vi "9202_conversions.vi"(11 "data":dbl[](array[numeric])) -> (3 "Array":dbl[](array[numeric]))   [LabVIEW 2019]
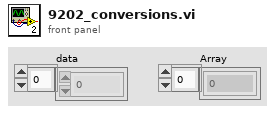
[diagram p1: front panel]
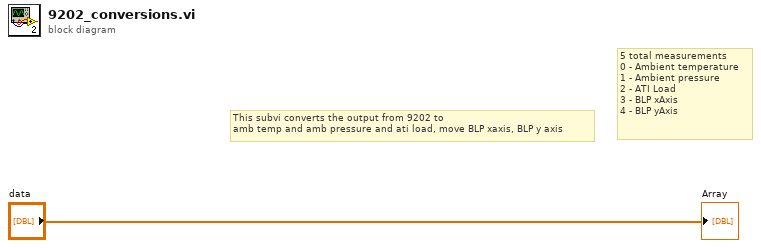
[diagram p0: block diagram]
diagram:
  # "5 total measurements\n0 - Ambient temperature\n1 - Ambient pressure\n2 - ATI Load\n3 - BLP xAxis\n4 - BLP yAxis"
  # "This subvi converts the output from 9202 to \namb temp and amb pressure and ati load, move BLP xaxis, BLP y axis"
  "Array" <- "data"
